vi "DynamicVIs.vi"   [LabVIEW 2016]
panel:
  # ">>> Include this VI in Builder!!! <<<"
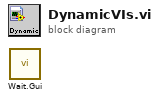
[diagram p0: block diagram]
diagram:
  n1 = call "Wait.Gui.vi"() -> ()  [unwired: 12 in]
